vi "Generate Chessboard Image Data (Regular).vi"(8 "error in (no error)":errorcluster, 10 "Chessboard Corners Info":T2, 11 "Target Size":T1) -> (0 "error out":errorcluster, 3 "Chessboard Image Data":u8[][](array[numeric]) format="%.0x")   [LabVIEW 2020, in "feature_detection.lvlib"]
doc: "Generate a chessboard for use with the Find Chessboard Corners Function and Camera Calibration."
uses:
  feature_detection.lvlib
  Chessboard Corner Info.ctl
  common/Image Size (Integer).ctl
  <vilib>/picture/pictutil.llb/Picture to Pixmap.vi
  <vilib>/picture/pixmap.llb/Unflatten Pixmap.vi
  common/common.lvlib
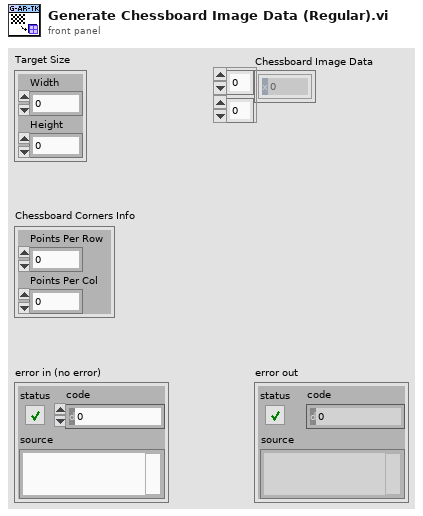
[diagram p1: front panel]
types:
  T1 = typedef "common.lvlib/Image Size (Integer).ctl" = cluster{"Width":u16, "Height":u16}
  T2 = typedef "feature_detection.lvlib/Chessboard Corner Info.ctl" = cluster{"Points Per Row":u8, "Points Per Col":u8}
  T3 = cluster{"Points Per Row":i32, "Points Per Col":i32}
  T4 = cluster{"left":i32, "top":i32, "right":i32, "bottom":i32}
  T5 = cluster{"Width":i16, "Style":enum32{"Solid", "Dash", "Dot", "DashDot", "DashDotDot"}}
  T6 = cluster{"left":i16, "top":i16, "right":i16, "bottom":i16}
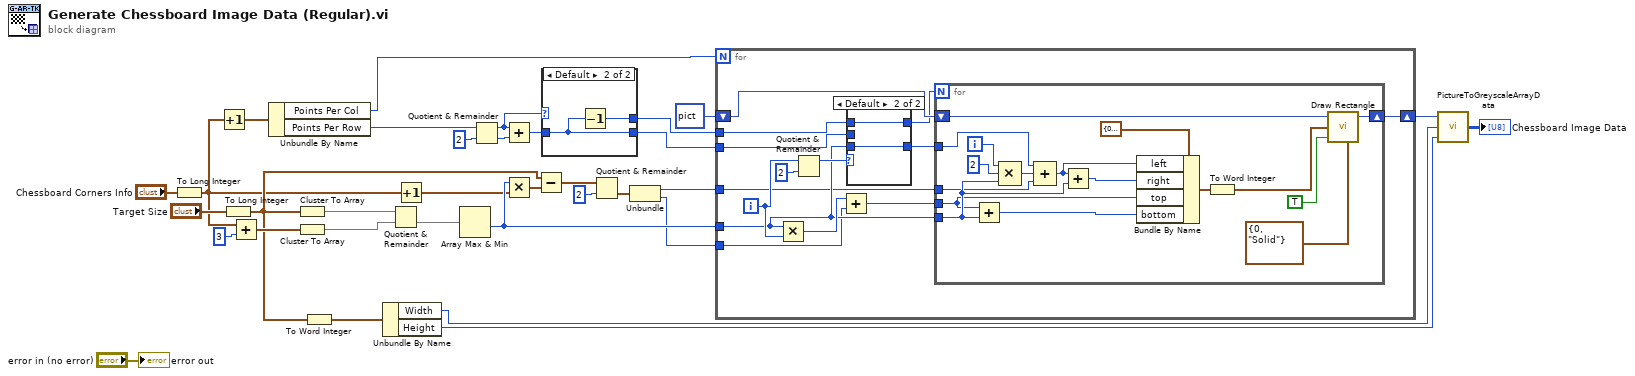
[diagram p0: block diagram]
diagram:
  n1 = To Long Integer(number="Chessboard Corners Info") -> (32bit integer=w4:T3)
  n2 = Increment(x=w4) -> (x+1=w27:T3)
  n3 = To Long Integer(number="Target Size") -> (32bit integer=w9:cluster{"Width":i32, "Height":i32})
  n4 = Add(x=w4, y=u16 3) -> (x+y=w18:T3)
  n5 = Unbundle By Name(w27) -> ("Points Per Col"=w25:i32, "Points Per Row"=w26:i32)
  n6 = Cluster To Array(cluster=w9) -> (array=w10:i32[])
  n7 = Cluster To Array(cluster=w18) -> (array=w11:i32[])
  n8 = To Word Integer(number=w9) -> (16bit integer=w17:cluster{"Width":i16, "Height":i16})
  n9 = Unbundle By Name(w17) -> ("Width"=w3:i16, "Height"=w2:i16)
  n10 = Quotient & Remainder(x=w10, y=w11) -> (floor(x/y)=w31:i32[])  [unwired: 1 out]
  n11 = Increment(x=w4) -> (x+1=w12:T3)
  n12 = Array Max & Min(array=w31) -> (min value=w19:i32)  [unwired: 3 out]
  n13 = Quotient & Remainder(x=w26, y=2) -> (x-y*floor(x/y)=w24:i32, floor(x/y)=w29:i32)
  n14 = Add(x=w24, y=w29) -> (x+y=w8:i32)
  n15 = Multiply(x=w19, y=w12) -> (x*y=w16:T3)
  n16 = Subtract(x=w9, y=w16) -> (x-y=w15:cluster{i32, i32})
  n17 = case shown="Default" w24 {
    tunnel: [w34 w35] -> w23
    tunnel: w8 -> [w34 w35]
    tunnel: [w34 w36] -> w22
    frame 0 {
    }
    frame Default {
      n18 = Decrement(x=w35) -> (x-1=w36:i32)
    }
  }
  n19 = Quotient & Remainder(x=w15, y=2) -> (floor(x/y)=w7:cluster{i32, i32})  [unwired: 1 out]
  n20 = Unbundle(w7) -> (w14:i32, w13:i32)
  n21 = for {
    N: w25 -> [_]
    shift-right: [w44] -> w21
    shift-left: picture data[5B] ("picture") -> [w50]
    tunnel: w23 -> [w42]
    tunnel: w19 -> [w39]
    tunnel: w22 -> [w41]
    tunnel: w14 -> [w38]
    tunnel: w13 -> [w37]
    i -> [w46]
    n22 = Multiply(x=w39, y=w46) -> (x*y=w45:i32)
    n23 = Quotient & Remainder(x=w46, y=2) -> (x-y*floor(x/y)=w48:i32)  [unwired: 1 out]
    n24 = Add(x=w45, y=w37) -> (x+y=w40:i32)
    n25 = case shown="Default" w48 {
      tunnel: w39 -> [_ w53]
      tunnel: [_ w53] -> w47
      tunnel: [w51 w52] -> w43
      tunnel: w42 -> [w51 _]
      tunnel: w41 -> [_ w52]
      frame 0 {
      }
      frame Default {
      }
    }
    n26 = for {
      N: w43 -> [_]
      tunnel: w39 -> [w59]
      shift-right: [w68] -> w44
      shift-left: w50 -> [w70]
      tunnel: w47 -> [w65]
      tunnel: w40 -> [w55]
      tunnel: w38 -> [w54]
      i -> [w64]
      n27 = Add(x=w55, y=w59) -> (x+y=w60:i32)
      n28 = Compound Arithmetic op=MULTIPLY(w64, 2 ("y"), w59) -> (w62:i32)
      n29 = Compound Arithmetic op=ADD(w65, w62, w54) -> (w61:i32)
      n30 = Add(x=w61, y=w59) -> (x+y=w56:i32)
      n31 = Bundle By Name(cluster=T4 {"left"=0, "top"=0, "right"=0, "bottom"=0} ("32bit integer"), "left"=w61, "right"=w56, "top"=w55, "bottom"=w60) -> (w69:T4)
      n32 = To Word Integer(number=w69) -> (16bit integer=w58:T6)
      n33 = call <vilib>:"Draw Rectangle.vi"("picture"=w70, "rect"=w58, "fill?(F)"=TRUE, "pen"=T5 {"Width"=0, "Style"=enum."Solid"}) -> ("new picture"=w68:picture)  [unwired: 5 in]
    }
  }
  n34 = call "PictureToGreyscaleArrayData.vi"("Bottom"=w2, "Right"=w3, "Picture"=w21) -> ("Greyscale Image Data"=→"Chessboard Image Data":u8[][])  [unwired: 2 in]
  "error out" <- "error in (no error)"
